vi "9205_Read_Mod4.vi"(10 "error in":errorcluster) -> (2 "error out":errorcluster, 3 "data out":fxp<+/-,26,5>[](array[numeric]))   [LabVIEW 2015]
uses:
  <vilib>/rvi/eio/common/nirviEmuTemplateMethod_errors.vi
  <vilib>/eio/EIONode/EIONode.xnode
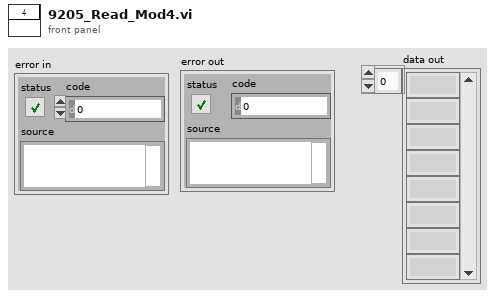
[diagram p1: front panel]
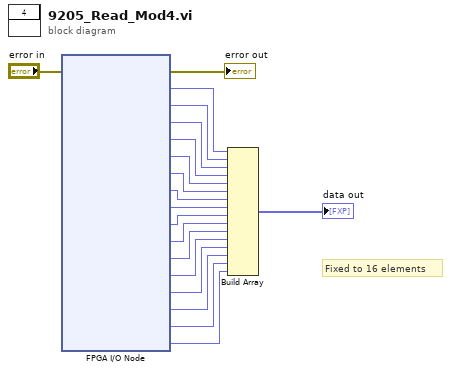
[diagram p0: block diagram]
diagram:
  # "Fixed to 16 elements"
  n1 = xnode "FPGA I/O Node"("error in"="error in") -> ("error out"=→"error out":errorcluster, "Mod4/AI0"=w7:fxp<+/-,26,5>, "Mod4/AI1"=w6:fxp<+/-,26,5>, "Mod4/AI2"=w5:fxp<+/-,26,5>, "Mod4/AI3"=w4:fxp<+/-,26,5>, "Mod4/AI4"=w19:fxp<+/-,26,5>, "Mod4/AI5"=w18:fxp<+/-,26,5>, "Mod4/AI6"=w17:fxp<+/-,26,5>, "Mod4/AI7"=w16:fxp<+/-,26,5>, "Mod4/AI16"=w15:fxp<+/-,26,5>, "Mod4/AI17"=w14:fxp<+/-,26,5>, "Mod4/AI18"=w13:fxp<+/-,26,5>, "Mod4/AI19"=w12:fxp<+/-,26,5>, "Mod4/AI20"=w11:fxp<+/-,26,5>, "Mod4/AI21"=w10:fxp<+/-,26,5>, "Mod4/AI22"=w9:fxp<+/-,26,5>, "Mod4/AI23"=w8:fxp<+/-,26,5>)  [unwired: 16 in, 16 out]
  n2 = Build Array(w7, w6, w5, w4, w19, w18, w17, w16, w15, w14, w13, w12, w11, w10, w9, w8) -> (→"data out":fxp<+/-,26,5>[])
